vi "Create menu items.vi"(8 "Error In":errorcluster, 11 "Menu ref in":refnum<k9>) -> (0 "Error Out":errorcluster, 3 "Menu ref out":refnum<k9>)   [LabVIEW 2015]
uses:
  <vilib>/Utility/miscctls.llb/LVMenuShortCut.ctl
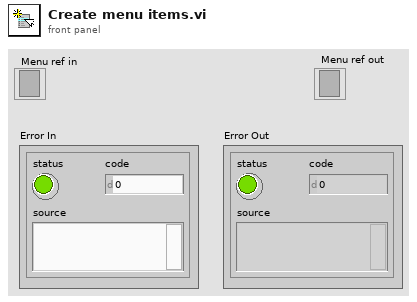
[diagram p1: front panel]
types:
  T1 = typedef "LVMenuShortCut.ctl" = cluster{"Include Shift Key?":bool, "Include Ctrl Key?":bool, "Shortcut Key":string}
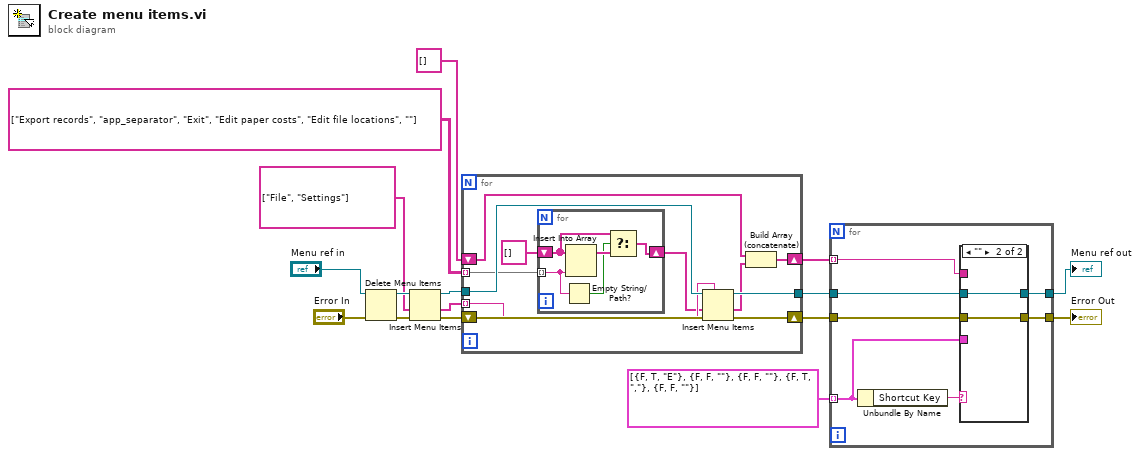
[diagram p0: block diagram]
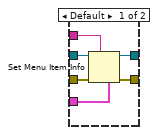
[diagram p2: hidden frame]
diagram:
  n1 = Delete Menu Items(6:"Error In", 9:"Menu ref in") -> (0:w16:errorcluster, 3:w15:refnum<k9>)  [unwired: 2 in]
  n2 = Insert Menu Items(6:w16, 7:string[] ["File", "Settings"], 9:w15) -> (0:w14:errorcluster, 1:w12:string[], 3:w13:refnum<k9>)  [unwired: 3 in]
  n3 = for {
    tunnel: w13 -> [w26]
    tunnel: w12 -> [w25] mode=indexing
    tunnel: string[][] [["Export records", "app_separator", "Exit"], ["Edit paper costs", "Edit file locations", ""]] -> [w23] mode=indexing
    tunnel: [w20] -> w6
    shift-right: [w21] -> w5
    shift-left: w14 -> [w27]
    shift-right: [w17] -> w4
    shift-left: string[] [] -> [w19]
    n4 = for {
      shift-right: [w31] -> w22
      shift-left: string[] [] -> [w30]
      tunnel: w23 -> [w28] mode=indexing
      n5 = Empty String/Path?(string/path=w28) -> (empty?=w29:bool)
      n6 = Insert Into Array(array=w30, new element=w28) -> (w32:string[])  [unwired: 1 in]
      n7 = Select(t=w30, s=w29, f=w32) -> (s? t:f=w31:string[])
    }
    n8 = Insert Menu Items(5:w25, 6:w27, 7:w22, 9:w26) -> (0:w21:errorcluster, 1:w18:string[], 3:w20:refnum<k9>)  [unwired: 2 in]
    n9 = Build Array (concatenate)(w19, w18) -> (w17:string[])
  }
  n10 = for {
    tunnel: w6 -> [w39]
    tunnel: w5 -> [w38]
    tunnel: w4 -> [w37] mode=indexing
    tunnel: T1[] [{"Include Shift Key?"=FALSE, "Include Ctrl Key?"=TRUE, "Shortcut Key"="E"}, {"Include Shift Key?"=FALSE, "Include Ctrl Key?"=FALSE, "Shortcut Key"=""}, {"Include Shift Key?"=FALSE, "Include Ctrl Key?"=FALSE, "Shortcut Key"=""}, {"Include Shift Key?"=FALSE, "Include Ctrl Key?"=TRUE, "Shortcut Key"=","}, {"Include Shift Key?"=FALSE, "Include Ctrl Key?"=FALSE, "Shortcut Key"=""}] ("short cut") -> [w34] mode=indexing
    tunnel: [w36] -> w2
    tunnel: [w35] -> w1
    n11 = Unbundle By Name(w34) -> ("Shortcut Key"=w33:string)
    n12 = case shown="\"\"" w33 {
      tunnel: w39 -> [w45 w47]
      tunnel: w38 -> [w44 w46]
      tunnel: w37 -> [w43 _]
      tunnel: w34 -> [w42 _]
      tunnel: [w41 w47] -> w36
      tunnel: [w40 w46] -> w35
      frame Default {
        n13 = Set Menu Item Info(4:w42, 7:w43, 8:w44, 11:w45) -> (0:w40:errorcluster, 3:w41:refnum<k9>)  [unwired: 3 in]
      }
      frame "" {
      }
    }
  }
  "Error Out" <- w1
  "Menu ref out" <- w2
